vi "mix_freq_array.vi"(9 "Freq Array In":dbl[](array[numeric]), 11 "Synth Controls":T1={"Channel Settings"=[{"Voltage (Amp.) "=6.0, "Frequency (MHz)"=0.0, "Phase (deg)"=0.0, "Nickname"="Blue MOT"}, {"Voltage (Amp.) "=9.0, "Frequency (MHz)"=0.0, "Phase (deg)"=0.0, "Nickname"="Hold"}, {"Voltage (Amp.) "=11.0, "Frequency (MHz)"=0.0, "Phase (deg)"=0.0, "Nickname"="Repump"}, {"Voltage (Amp.) "=10.0, "Frequency (MHz)"=0.0, "Phase (deg)"=0.0, "Nickname"="Red MOT"}, {"Voltage (Amp.) "=11.0, "Frequency (MHz)"=0.0, "Phase (deg)"=0.0, "Nickname"="Load ODT"}, {"Voltage (Amp.) "=11.0, "Frequency (MHz)"=0.0, "Phase (deg)"=0.0, "Nickname"="ODT Hold"}, {"Voltage (Amp.) "=11.0, "Frequency (MHz)"=0.0, "Phase (deg)"=0.0, "Nickname"=""}, {"Voltage (Amp.) "=200.0, "Frequency (MHz)"=2.0, "Phase (deg)"=0.0, "Nickname"="loop hold"}, {"Voltage (Amp.) "=0.0, "Frequency (MHz)"=0.0, "Phase (deg)"=0.0, "Nickname"=""}, {"Voltage (Amp.) "=0.0, "Frequency (MHz)"=0.0, "Phase (deg)"=0.0, "Nickname"="expose uv"}, {"Voltage (Amp.) "=7.0, "Frequency (MHz)"=3.0, "Phase (deg)"=0.0, "Nickname"=""}, {"Voltage (Amp.) "=0.0, "Frequency (MHz)"=0.0, "Phase (deg)"=0.0, "Nickname"="Drop"}, {"Voltage (Amp.) "=0.0, "Frequency (MHz)"=0.0, "Phase (deg)"=0.0, "Nickname"="Image atoms "}, {"Voltage (Amp.) "=0.0, "Frequency (MHz)"=0.0, "Phase (deg)"=0.0, "Nickname"="Wait"}, {"Voltage (Amp.) "=0.0, "Frequency (MHz)"=0.0, "Phase (deg)"=0.0, "Nickname"="Image BG"}, {"Voltage (Amp.) "=0.0, "Frequency (MHz)"=6.0, "Phase (deg)"=0.0, "Nickname"="Kill time"}], "Active Chans"=[TRUE, FALSE, FALSE, FALSE], "COM Port"="COM5", "Table Mode"={"Initial Freq.(MHz)"=0.0, "FinalFreq"=0.0, "Freq. Step (MHz)"=0.0, "Voltage (Amp.)"=0.0, "Asc. & Desc."=FALSE, "Custom Frequencies"=[], "Custom Amplitude"=[], "Table Mode Switch"=FALSE, "Array Gen"=enum."Auto", "Randomize"=FALSE, "Continuous"=FALSE}} {"Table Mode"."Freq. Step (MHz)" format="%#_9g"; "Table Mode"."FinalFreq" format="%#_9g"; "Table Mode"."Initial Freq.(MHz)" format="%#_9g"; "Channel Settings"."Frequency (MHz)" format="%#_9g"}) -> (1 "Mixed Freq Array":dbl[](array[numeric]), 3 "Synth Controls Out":T1={"Channel Settings"=[{"Voltage (Amp.) "=6.0, "Frequency (MHz)"=0.0, "Phase (deg)"=0.0, "Nickname"="Blue MOT"}, {"Voltage (Amp.) "=9.0, "Frequency (MHz)"=0.0, "Phase (deg)"=0.0, "Nickname"="Hold"}, {"Voltage (Amp.) "=11.0, "Frequency (MHz)"=0.0, "Phase (deg)"=0.0, "Nickname"="Repump"}, {"Voltage (Amp.) "=10.0, "Frequency (MHz)"=0.0, "Phase (deg)"=0.0, "Nickname"="Red MOT"}, {"Voltage (Amp.) "=11.0, "Frequency (MHz)"=0.0, "Phase (deg)"=0.0, "Nickname"="Load ODT"}, {"Voltage (Amp.) "=11.0, "Frequency (MHz)"=0.0, "Phase (deg)"=0.0, "Nickname"="ODT Hold"}, {"Voltage (Amp.) "=11.0, "Frequency (MHz)"=0.0, "Phase (deg)"=0.0, "Nickname"=""}, {"Voltage (Amp.) "=200.0, "Frequency (MHz)"=2.0, "Phase (deg)"=0.0, "Nickname"="loop hold"}, {"Voltage (Amp.) "=0.0, "Frequency (MHz)"=0.0, "Phase (deg)"=0.0, "Nickname"=""}, {"Voltage (Amp.) "=0.0, "Frequency (MHz)"=0.0, "Phase (deg)"=0.0, "Nickname"="expose uv"}, {"Voltage (Amp.) "=7.0, "Frequency (MHz)"=3.0, "Phase (deg)"=0.0, "Nickname"=""}, {"Voltage (Amp.) "=0.0, "Frequency (MHz)"=0.0, "Phase (deg)"=0.0, "Nickname"="Drop"}, {"Voltage (Amp.) "=0.0, "Frequency (MHz)"=0.0, "Phase (deg)"=0.0, "Nickname"="Image atoms "}, {"Voltage (Amp.) "=0.0, "Frequency (MHz)"=0.0, "Phase (deg)"=0.0, "Nickname"="Wait"}, {"Voltage (Amp.) "=0.0, "Frequency (MHz)"=0.0, "Phase (deg)"=0.0, "Nickname"="Image BG"}, {"Voltage (Amp.) "=0.0, "Frequency (MHz)"=6.0, "Phase (deg)"=0.0, "Nickname"="Kill time"}], "Active Chans"=[TRUE, FALSE, FALSE, FALSE], "COM Port"="COM5", "Table Mode"={"Initial Freq.(MHz)"=0.0, "FinalFreq"=0.0, "Freq. Step (MHz)"=0.0, "Voltage (Amp.)"=0.0, "Asc. & Desc."=FALSE, "Custom Frequencies"=[], "Custom Amplitude"=[], "Table Mode Switch"=FALSE, "Array Gen"=enum."Auto", "Randomize"=FALSE, "Continuous"=FALSE}} {"Table Mode"."Freq. Step (MHz)" format="%#_9g"; "Table Mode"."FinalFreq" format="%#_9g"; "Table Mode"."Initial Freq.(MHz)" format="%#_9g"; "Channel Settings"."Frequency (MHz)" format="%#_9g"})   [LabVIEW 2016]
uses:
  Controls/Synth_409b/Synth_controls.ctl
  Controls/Synth_409b/synth_channel.ctl
  Controls/Synth_409b/table_mode.ctl
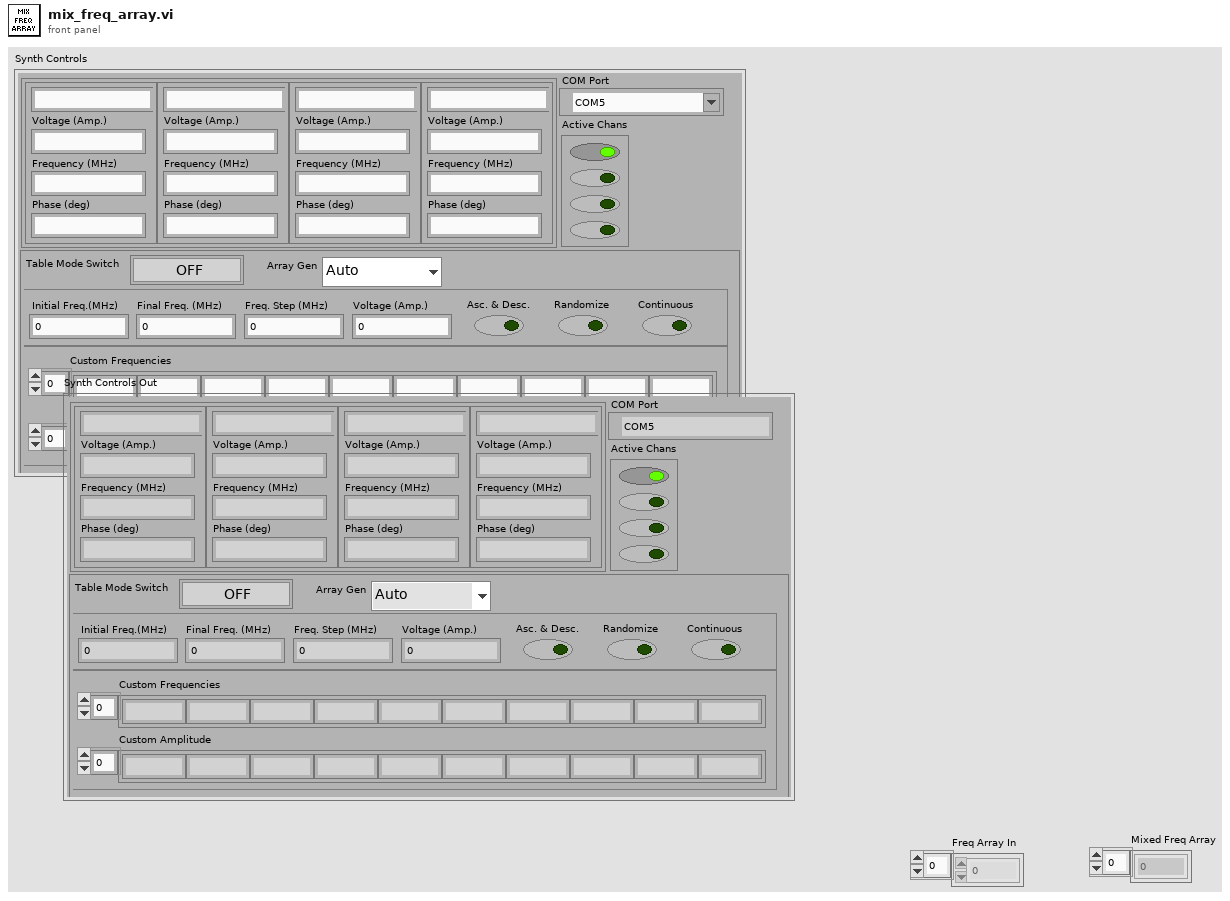
[diagram p1: front panel]
types:
  T1 = typedef "Synth_controls.ctl" = cluster{"Channel Settings":T2[], "Active Chans":bool[], "COM Port":refnum<visa-resource-name>, "Table Mode":T3}
  T2 = typedef "synth_channel.ctl" = cluster{"Voltage (Amp.) ":dbl, "Frequency (MHz)":dbl, "Phase (deg)":dbl, "Nickname":string}
  T3 = typedef "table_mode.ctl" = cluster{"Initial Freq.(MHz)":dbl, "FinalFreq":dbl, "Freq. Step (MHz)":dbl, "Voltage (Amp.)":dbl, "Asc. & Desc.":bool, "Custom Frequencies":dbl[], "Custom Amplitude":dbl[], "Table Mode Switch":bool, "Array Gen":enum16{"Auto", "Custom"}, "Randomize":bool, "Continuous":bool}
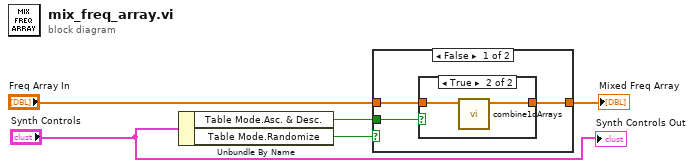
[diagram p0: block diagram]
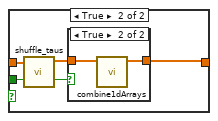
[diagram p3: hidden frame]
diagram:
  n1 = Unbundle By Name("Synth Controls") -> ("Table Mode.Asc. & Desc."=w1:bool, "Table Mode.Randomize"=w5:bool)
  n2 = case shown="False" w5 {
    tunnel: "Freq Array In" -> [w8 w15]
    tunnel: [w7 w13] -> w3
    tunnel: w1 -> [w6 w12]
    frame False {
      n3 = case shown="True" w6 {
        tunnel: w8 -> [w9 w11]
        tunnel: [w9 w10] -> w7
        frame False {
        }
        frame True {
          n4 = call "combine1dArrays.vi"("Array In"=w11) -> ("Array Out"=w10:dbl[])  [unwired: 10 in]
        }
      }
    }
    frame True {
      n5 = call "shuffle_taus.vi"("Array In"=w15) -> ("Mixed Array Out"=w14:dbl[])  [unwired: 10 in]
      n6 = case shown="True" w12 {
        tunnel: w14 -> [w16 w18]
        tunnel: [w16 w17] -> w13
        frame False {
        }
        frame True {
          n7 = call "combine1dArrays.vi"("Array In"=w18) -> ("Array Out"=w17:dbl[])  [unwired: 10 in]
        }
      }
    }
  }
  "Mixed Freq Array" <- w3
  "Synth Controls Out" <- "Synth Controls"
